vi "1-Exp Decay Parameters from Gated Decay.vi"(6 "Gate Width: W":dbl, 7 "period: T":dbl, 8 "# Gates":dbl, 9 "Min Decay":dbl, 10 "Mid Decay":dbl, 11 "Max Decay":dbl) -> (0 "I":dbl, 1 "x":dbl, 2 "tau":dbl, 3 "B":dbl)   [LabVIEW 2019]
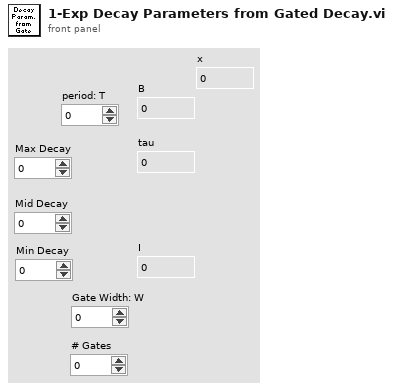
[diagram p1: front panel]
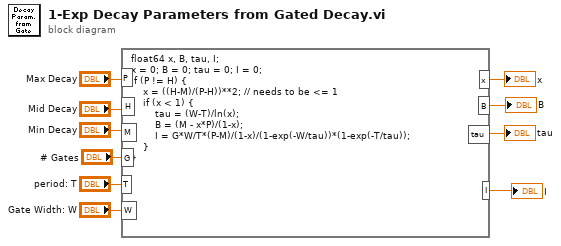
[diagram p0: block diagram]
diagram:
  n1 = formula code="float64 x, B, tau, I;\nx = 0; B = 0; tau = 0; I = 0;\nif (P != H) {\n    x = ((H-M)/(P-H))**2; // needs to be <= 1\n    if (x < 1) {\n        tau = (W-T)/ln(x);\n        B = (M - x*P)/(1-x);\n        I = G*W/T*(P-M)/(1-x)/(1-exp(-W/tau))*(1-exp(-T/tau));\n    }\n}"("T"="period: T", "W"="Gate Width: W", "P"="Max Decay", "M"="Min Decay", "H"="Mid Decay", "G"="# Gates") -> ("tau"=→"tau":dbl, "B"=→"B":dbl, "x"=→"x":dbl, "I"=→"I":dbl)
